vi "Circular Buffer (BRAM) _U128.vi"(7 "Buffer Pointers":T2, 8 "Input Valid":bool, 9 "Read Data?":bool, 10 "Start Buffering":bool, 11 "Input Write Data":T1) -> (0 "Output Valid":bool, 3 "Output Write Data":T1)   [LabVIEW 2011]
doc: "This VI maintains a circular buffer with user configurable buffer size.\nMaximum Buffer Size = 4096 (U32) elements\n\n<b> Delay = 1 Tick </b>"
uses:
  <vilib>/rvi/DataTransferAndStorage/Container/Common/niFpgaContainerState.ctl
  <vilib>/rvi/DataTransferAndStorage/Container/Common/niFpgaDataTypeControl.ctl
  <vilib>/rvi/DataTransferAndStorage/Container/Common/niFpgaContainerImplementationControl.ctl
  <vilib>/rvi/DataTransferAndStorage/Container/Common/niFpgaContainerArbitrationOptionsControl.ctl
  <vilib>/rvi/DataTransferAndStorage/Container/Common/niFpgaTransferTypeControl.ctl
  <vilib>/rvi/DataTransferAndStorage/Container/Common/niFpgaContainerInitializationParameters.ctl
  <vilib>/rvi/Memory/Memory_Types/niFpgaMemoryInterfaceConfiguration.ctl
  <vilib>/rvi/FIFO/Fifo_Types/niFpgaFifoControlLogicControl.ctl
  <vilib>/rvi/DataTransferAndStorage/Container/Common/niFpgaContainerMetaDataKey.ctl
  <vilib>/rvi/DataTransferAndStorage/Container/Common/niFpgaContainerGetUniqueNameForEmu.vi
  <vilib>/rvi/DataTransferAndStorage/Container/Common/niFpgaContainerSetEmuInfo.vi
  <vilib>/rvi/eio/common/nirviEmuReportErrorAndStop.vi
  <vilib>/rvi/Memory/Memory_Emulation/niFpgaMemoryEmulationValidateCache.vi
  <vilib>/rvi/Memory/Memory_Emulation/nirvimemoryEmulationManagerCache_InsertValue.vi
  <vilib>/Utility/error.llb/Clear Errors.vi
  <vilib>/rvi/Memory/Memory_Emulation/nirvimemoryEmulationManagerCache_GetValue.vi
  <vilib>/rvi/Memory/Memory_Emulation/nirvimemoryEmulationManagerCache_SetValue.vi
  <vilib>/rvi/LocalResourceManager/LocalResourceManager.xnode
  <vilib>/rvi/DataTransferAndStorage/Container/XNode/niFpgaContainer.xnode
  <vilib>/rvi/Memory/Memory_Emulation/nirvimemoryEmulation.vi
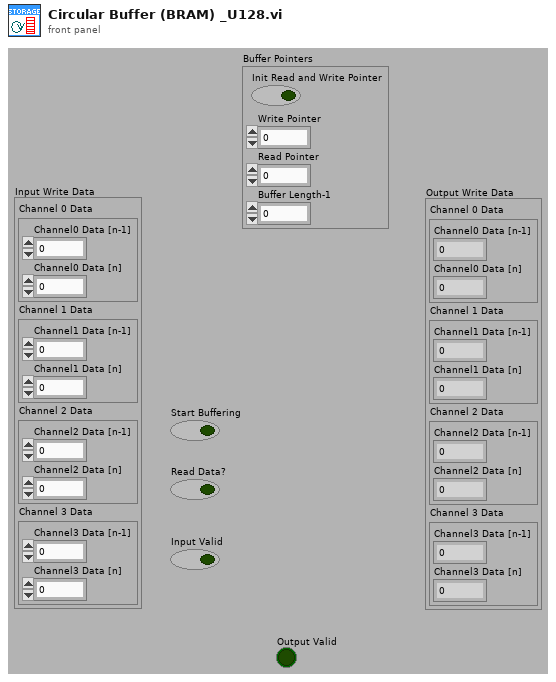
[diagram p1: front panel]
types:
  T1 = cluster{"Channel 0 Data":cluster{"Channel0 Data [n-1]":i16, "Channel0 Data [n]":i16}, "Channel 1 Data":cluster{"Channel1 Data [n-1]":i16, "Channel1 Data [n]":i16}, "Channel 2 Data ":cluster{"Channel2 Data [n-1]":i16, "Channel2 Data [n]":i16}, "Channel 3 Data":cluster{"Channel3 Data [n-1]":i16, "Channel3 Data [n]":i16}}
  T2 = cluster{"Init Read and Write Pointer":bool, "Write Pointer":u16, "Read Pointer":u16, "Buffer Length-1":u16}
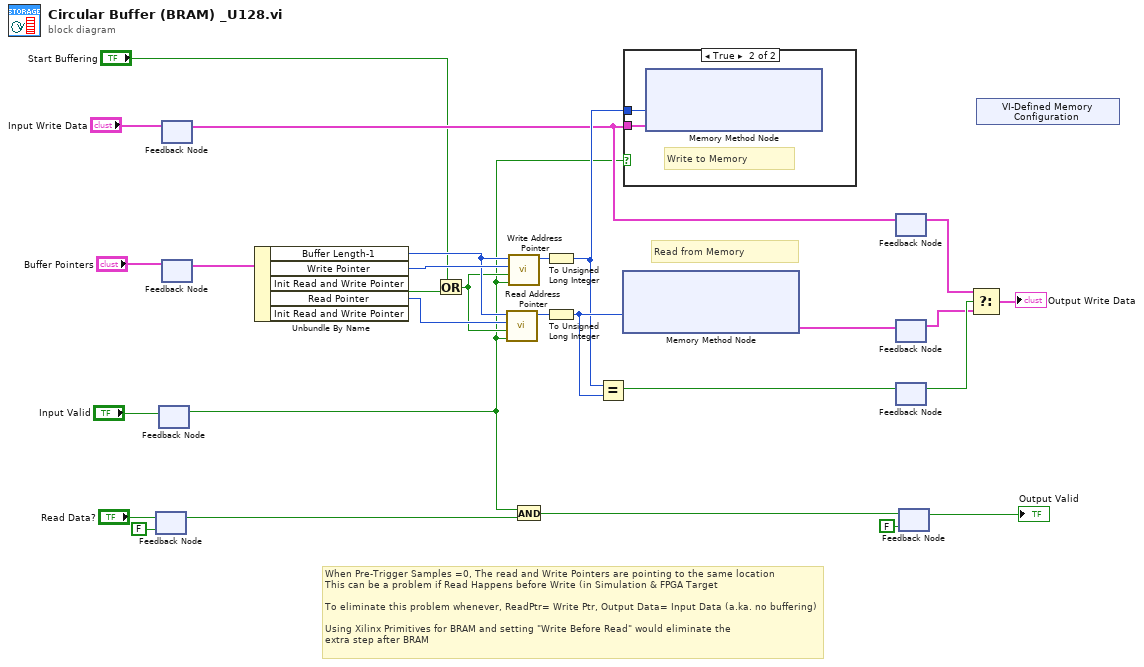
[diagram p0: block diagram]
diagram:
  # "When Pre-Trigger Samples =0, The read and Write Pointers are pointing to the same location\nThis can be a problem if Read Happens before Write (in Simulation & FPGA Target\n\nTo eliminate this problem whenever, ReadPtr= Write Ptr, Output Data= Input Data (a.ka. no buffering)\n\nUsing Xilinx Primitives for BRAM and setting \"Write Before Read\" would eliminate the\nextra step after BRAM"
  # "Read from Memory"
  n1 = feedback-in #1("Read Data?") -> ()
  n2 = feedback #1(FALSE ("Read Data?")) -> (w3:bool)
  n3 = feedback #2() -> (w4:bool)  [unwired: 1 in]
  n4 = feedback-in #2("Input Valid") -> ()
  n5 = feedback #3() -> (w12:T1)  [unwired: 1 in]
  n6 = feedback-in #3("Input Write Data") -> ()
  n7 = feedback #4() -> (w27:T2)  [unwired: 1 in]
  n8 = feedback-in #4("Buffer Pointers") -> ()
  n9 = Unbundle By Name(w27) -> ("Buffer Length-1"=w19:u16, "Write Pointer"=w21:u16, "Init Read and Write Pointer"=w8:bool, "Read Pointer"=w20:u16)  [unwired: 1 out]
  n10 = Or(x="Start Buffering", y=w8) -> (x .or. y?=w7:bool)
  n11 = call <userlib>:"Read Address Pointer.vi"("INC?"=w4, "Load?"=w7, "Load Value"=w20, "rollover"=w19) -> ("count"=w6:u16)  [unwired: 7 in]
  n12 = call <userlib>:"Write Address Pointer.vi"("INC?"=w4, "Load?"=w7, "Load Value"=w21, "rollover"=w19) -> ("count"=w5:u16)  [unwired: 7 in]
  n13 = And(x=w4, y=w3) -> (x .and. y?=w2:bool)
  n14 = To Unsigned Long Integer(number=w5) -> (unsigned 32bit integer=w15:u32)
  n15 = To Unsigned Long Integer(number=w6) -> (unsigned 32bit integer=w18:u32)
  n16 = Equal?(x=w15, y=w18) -> (x = y?=w16:bool)
  n17 = xnode ("Memory Method Node")("Address"=w18) -> ("Data"=w28:T1)  [unwired: 1 in, 1 out]
  n18 = case shown="True" w4 {
    tunnel: w12 -> [_ w30]
    tunnel: w15 -> [_ w29]
    frame False {
    }
    frame True {
      # "Write to Memory"
      n19 = xnode ("Memory Method Node")("Address"=w29, "Data"=w30) -> ()  [unwired: 1 in, 1 out]
    }
  }
  n20 = feedback #5() -> (w14:T1)  [unwired: 1 in]
  n21 = feedback-in #5(w12) -> ()
  n22 = feedback #6() -> (w13:T1)  [unwired: 1 in]
  n23 = feedback-in #6(w28) -> ()
  n24 = feedback #7() -> (w17:bool)  [unwired: 1 in]
  n25 = feedback-in #7(w16) -> ()
  n26 = feedback #8(FALSE ("Retrieve Data")) -> (→"Output Valid":bool)
  n27 = feedback-in #8(w2) -> ()
  n28 = Select(t=w14, s=w17, f=w13) -> (s? t:f=→"Output Write Data":T1)
  n29 = xnode "VI-Defined Memory Configuration"() -> ()  [unwired: 1 out]
